vi "DrawBrowseButtonDecal.vi"(11 "Size":cluster{"x":i32, "y":i32}={"x"=20, "y"=122}) -> (3 "image":T1)   [LabVIEW 2014, in "Raspberry Pi Compatible Compiler for LabVIEW.lvlib" / "Path.lvclass"]
uses:
  Path.lvclass
  <vilib>/picture/picture.llb/imagedata.ctl
  Raspberry Pi Compatible Compiler for LabVIEW.lvlib
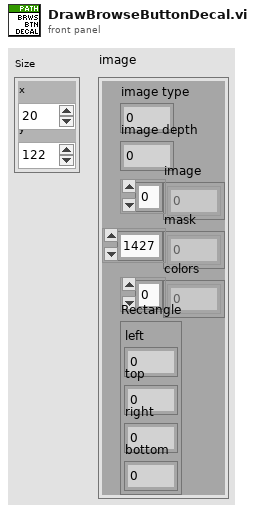
[diagram p1: front panel]
types:
  T1 = typedef "imagedata.ctl" = cluster{"image type":i32, "image depth":i32, "image":u8[], "mask":u8[], "colors":u32[], "Rectangle":cluster{"left":i16, "top":i16, "right":i16, "bottom":i16}}
  T2 = cluster{"left":i16, "top":i16, "right":i16, "bottom":i16}
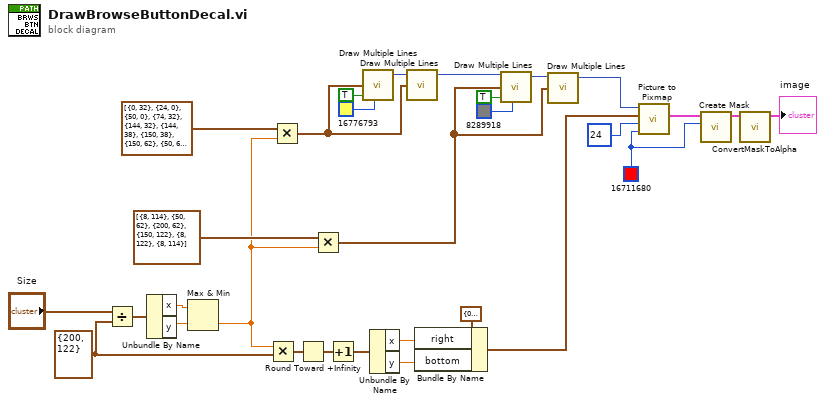
[diagram p0: block diagram]
diagram:
  w16 = u32 16711680 ("Background Color")
  w10 = cluster{"x":i32, "y":i32} {"x"=200, "y"=122}
  n1 = Divide(x="Size", y=w10) -> (x/y=w23:cluster{"x":dbl, "y":dbl})
  n2 = Unbundle By Name(w23) -> ("x"=w22:dbl, "y"=w21:dbl)
  n3 = Max & Min(x=w22, y=w21) -> (min(x,y)=w11:dbl)  [unwired: 1 out]
  n4 = Multiply(x=w11, y=w10) -> (x*y=w9:cluster{"x":dbl, "y":dbl})
  n5 = Multiply(x=cluster{"x":i16, "y":i16}[] [{"x"=0, "y"=32}, {"x"=24, "y"=0}, {"x"=50, "y"=0}, {"x"=74, "y"=32}, {"x"=144, "y"=32}, {"x"=144, "y"=38}, {"x"=150, "y"=38}, {"x"=150, "y"=62}, {"x"=50, "y"=62}, {"x"=8, "y"=114}, {"x"=0, "y"=114}, {"x"=0, "y"=32}] ("line endpoints"), y=w11) -> (x*y=w12:cluster{"x":dbl, "y":dbl}[])
  n6 = Round Toward +Infinity(x=w9) -> (ceil(x): smallest int >= x=w4:cluster{"x":dbl, "y":dbl})
  n7 = Multiply(x=cluster{"x":i16, "y":i16}[] [{"x"=8, "y"=114}, {"x"=50, "y"=62}, {"x"=200, "y"=62}, {"x"=150, "y"=122}, {"x"=8, "y"=122}, {"x"=8, "y"=114}] ("line endpoints"), y=w11) -> (x*y=w13:cluster{"x":dbl, "y":dbl}[])
  n8 = Increment(x=w4) -> (x+1=w3:cluster{"x":dbl, "y":dbl})
  n9 = call <vilib>:"Draw Multiple Lines.vi"("line endpoints"=w12, "fill?(F)"=TRUE, "color(black)"=u32 16776793) -> ("new picture"=w28:picture)  [unwired: 6 in]
  n10 = Unbundle By Name(w3) -> ("x"=w8:dbl, "y"=w6:dbl)
  n11 = call <vilib>:"Draw Multiple Lines.vi"("picture"=w28, "line endpoints"=w12) -> ("new picture"=w27:picture)  [unwired: 7 in]
  n12 = Bundle By Name(cluster=T2 {"left"=0, "top"=0, "right"=0, "bottom"=0} ("rect"), "right"=w8, "bottom"=w6) -> (w5:T2)
  n13 = call <vilib>:"Draw Multiple Lines.vi"("picture"=w27, "line endpoints"=w13, "fill?(F)"=TRUE, "color(black)"=u32 8289918) -> ("new picture"=w24:picture)  [unwired: 5 in]
  n14 = call <vilib>:"Draw Multiple Lines.vi"("picture"=w24, "line endpoints"=w13) -> ("new picture"=w18:picture)  [unwired: 7 in]
  n15 = call <vilib>:"Picture to Pixmap.vi"("Background Color"=w16, "depth"=24, "rect"=w5, "picture"=w18) -> ("image data"=w15:T1)  [unwired: 6 in, 1 out]
  n16 = call <vilib>:"Create Mask.vi"("Mask Color (Black)"=w16, "image data"=w15) -> ("image data"=w14:T1)  [unwired: 9 in]
  n17 = call "ConvertMaskToAlpha.vi"("input cluster"=w14) -> ("output cluster"=→"image":T1)  [unwired: 10 in]
